vi "Teleop_Dash_Write.vi"   [LabVIEW 2019]
uses:
  Teleop_Globals.vi
  <vilib>/Rock Robotics/Network Tables/NT Write Numeric Array.vi
  <vilib>/Rock Robotics/Network Tables/NT Write Boolean Array.vi
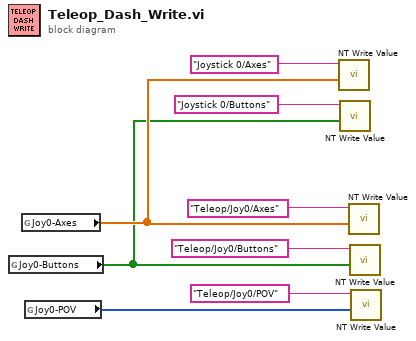
[diagram p0: block diagram]
diagram:
  n1 = global read "Teleop_Globals.vi" "Joy0-Buttons"() -> (w2:bool[])
  n2 = global read "Teleop_Globals.vi" "Joy0-Axes"() -> (w3:dbl[])
  n3 = global read "Teleop_Globals.vi" "Joy0-POV"() -> (w1:i32[])
  n4 = call-poly <vilib>:"NT Write Value.vi"("Numeric Array"=w3, "Name"="Joystick 0/Axes") -> ()  [unwired: 9 in, 1 out]
  n5 = call-poly <vilib>:"NT Write Value.vi"("Boolean Array"=w2, "Name"="Joystick 0/Buttons") -> ()  [unwired: 9 in, 1 out]
  n6 = call-poly <vilib>:"NT Write Value.vi"("Numeric Array"=w3, "Name"="Teleop/Joy0/Axes") -> ()  [unwired: 9 in, 1 out]
  n7 = call-poly <vilib>:"NT Write Value.vi"("Boolean Array"=w2, "Name"="Teleop/Joy0/Buttons") -> ()  [unwired: 9 in, 1 out]
  n8 = call-poly <vilib>:"NT Write Value.vi"("Numeric Array"=w1, "Name"="Teleop/Joy0/POV") -> ()  [unwired: 9 in, 1 out]
